vi "Get Log Entries.vi"(8 "error in (no error)":errorcluster, 11 "Server in":refnum<class "Server.lvclass">) -> (0 "error out":errorcluster, 2 "Log Entries":T1[](array[typedef]) {"Time Stamp" format="%<%y/%m/%d-%H:%M:%S%3u>T"}, 3 "Server out":refnum<class "Server.lvclass">)   [LabVIEW 2020, in "HTTP Server.lvlib" / "Server.lvclass"]
uses:
  Server.lvclass
  Access Log Entry.ctl
  Server.lvclass/Server.ctl
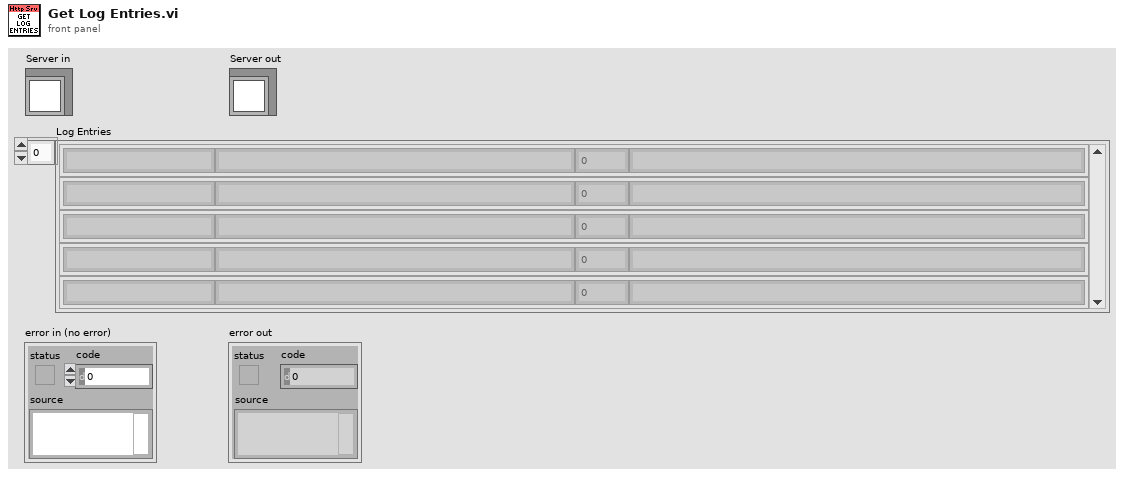
[diagram p1: front panel]
types:
  T1 = typedef "HTTP Server.lvlib/Server.lvclass/Access Log Entry.ctl" = cluster{"Time Stamp":timestamp, "Client":string, "Code":u16, "Info":string}
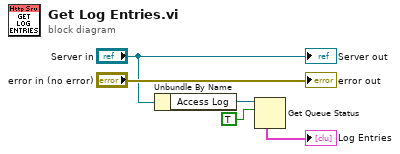
[diagram p0: block diagram]
diagram:
  n1 = Unbundle By Name("Server in") -> ("Access Log"=w3:refnum<queue>)
  n2 = Get Queue Status(queue=w3, return elements? (F)=TRUE) -> (elements=→"Log Entries":T1[])  [unwired: 1 in, 7 out]
  "error out" <- "error in (no error)"
  "Server out" <- "Server in"
